vi "Operate_CSM_template_doc.vi"(6 "Save to md(F)/Load to vi(T)":bool=TRUE, 9 "Path":path=path "D:/github/JKI-State-Machine-Plus/src/help/NEVSTOP/JKI State Machine++/Template Description.md", 11 "vi path":path=path "D:/github/JKI-State-Machine-Plus/src/user.lib/_NEVSTOP/JKI State Machine++/JKISM++ No-Event Structure Template.vi") -> ()   [LabVIEW 2014]
panel:
  out "Array":cluster{refnum<vi>, "Text":string}[](array[cluster])
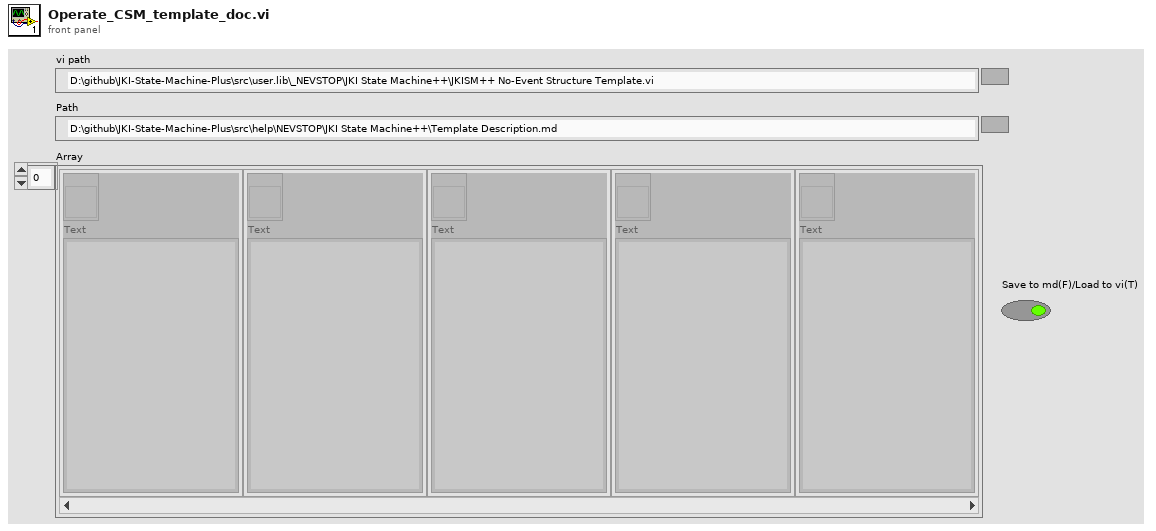
[diagram p1: front panel]
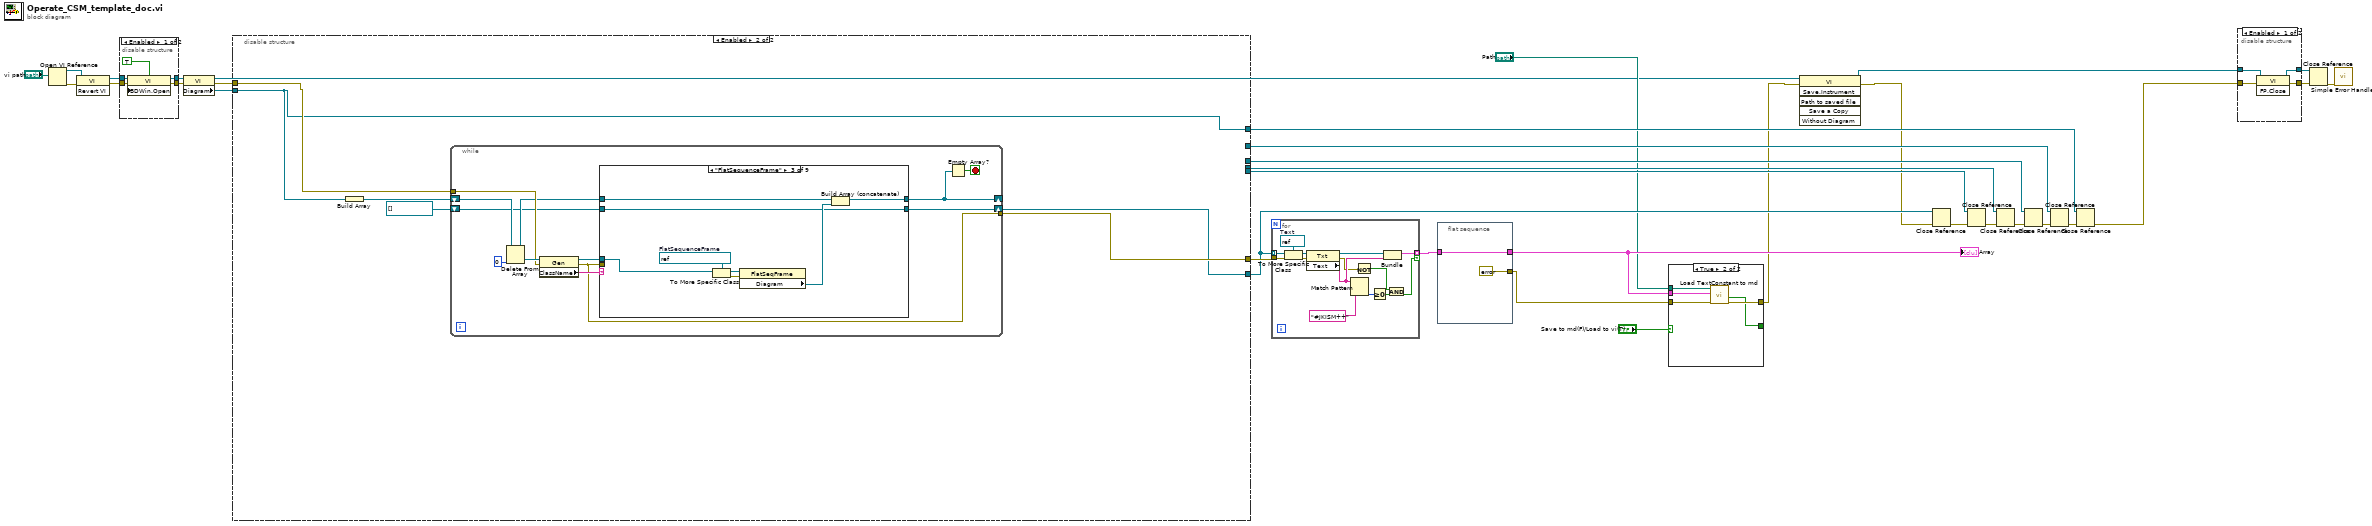
[diagram p0: block diagram]
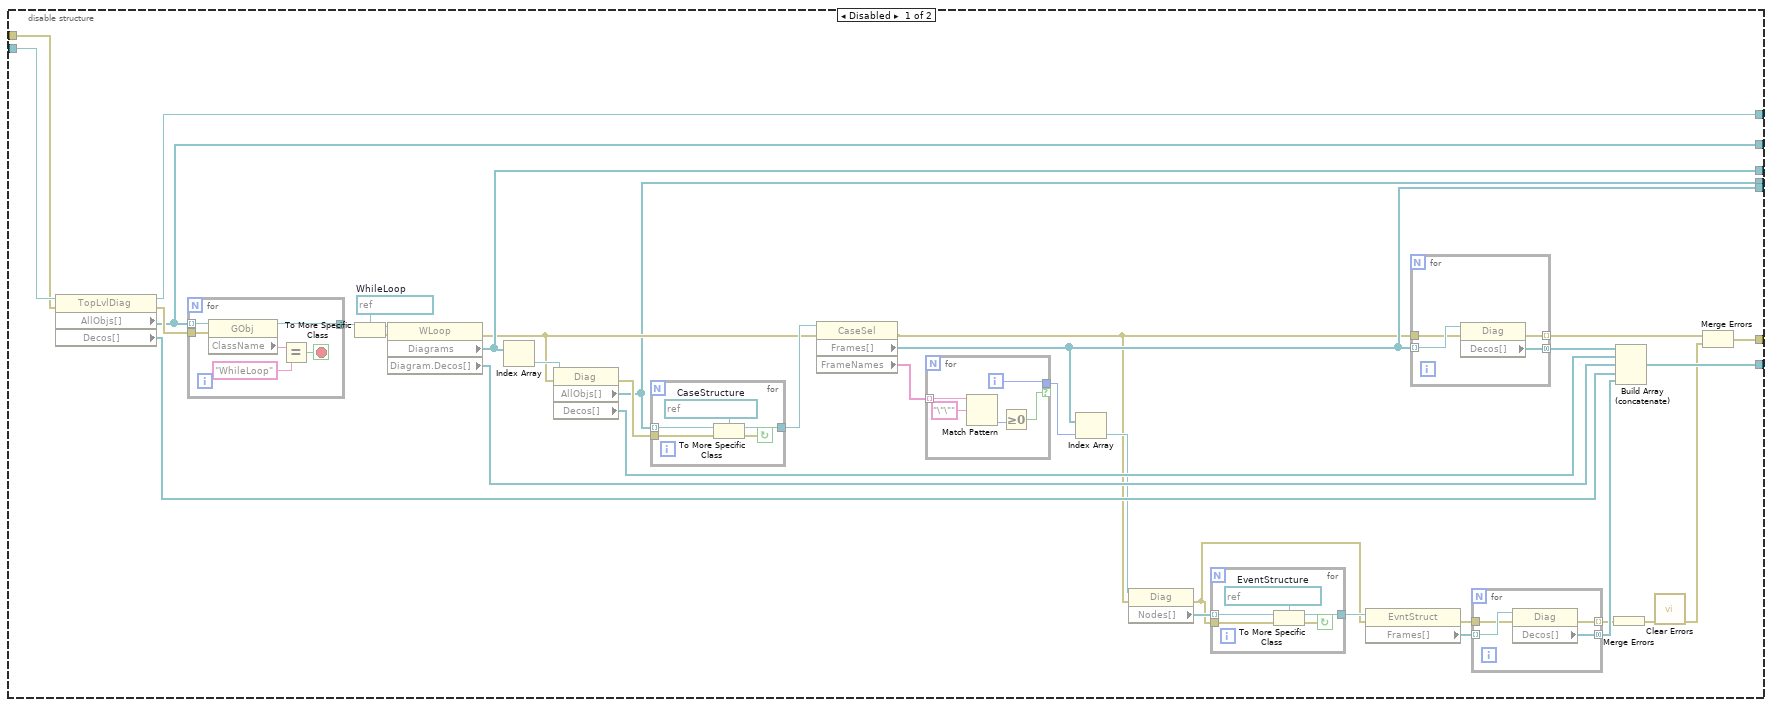
[diagram p2: hidden frame]
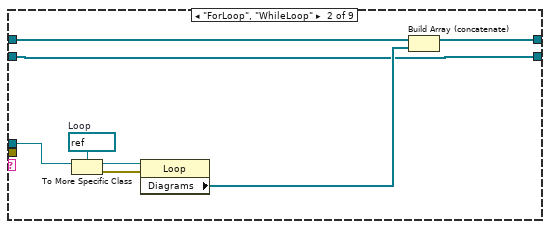
[diagram p4: hidden frame]
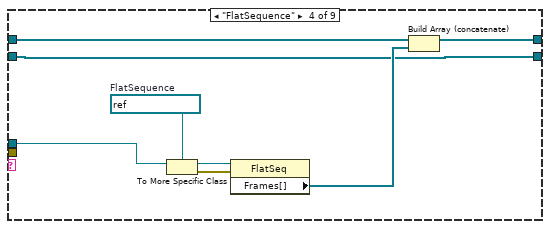
[diagram p5: hidden frame]
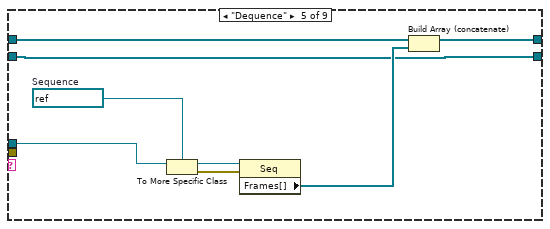
[diagram p6: hidden frame]
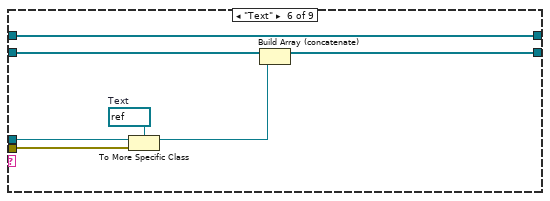
[diagram p7: hidden frame]
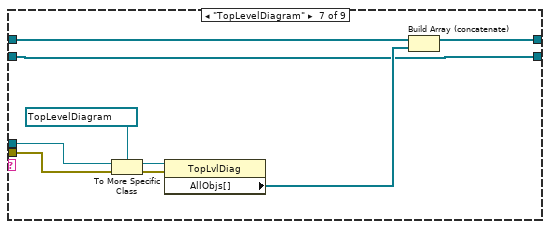
[diagram p8: hidden frame]
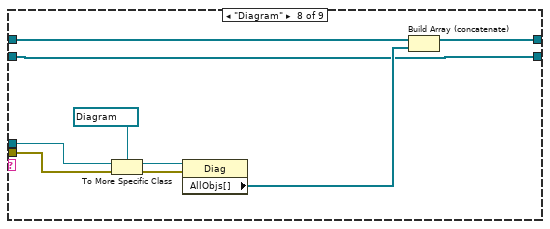
[diagram p9: hidden frame]
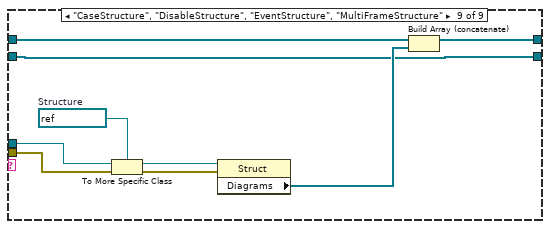
[diagram p10: hidden frame]
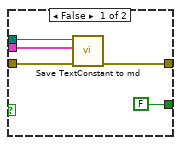
[diagram p12: hidden frame]
diagram:
  n1 = Open VI Reference(vi path="vi path") -> (vi reference=w33:refnum<vi>, error out=w34:errorcluster)  [unwired: 5 in]
  n2 = invoke class="VI" method="Revert VI"(reference=w33, error in=w34) -> (reference out=w25:refnum<vi>, error out=w24:errorcluster)  [unwired: 1 in, 1 out]
  n3 = disable-structure shown="Enabled" {
    disable-tunnel: w25 -> [w39 w41]
    disable-tunnel: w24 -> [w38 w40]
    disable-tunnel: [w37 w41] -> w23
    disable-tunnel: [w36 w40] -> w22
    frame Enabled {
      n4 = property class="VI"(reference=w39, error in=w38, "BDWin.Open"=TRUE ("Block Diagram Window:Open")) -> (reference out=w37:refnum<vi>, error out=w36:errorcluster)
    }
    frame Disabled {
    }
  }
  n5 = property class="VI"(reference=w23, error in=w22) -> (reference out=w4:refnum<vi>, error out=w30:errorcluster, "Diagram"=w31:refnum<vi>)
  n6 = disable-structure shown="Enabled" {
    disable-tunnel: w31 -> [w77 w107]
    disable-tunnel: w30 -> [w76 w110]
    disable-tunnel: [w70 _] -> w28
    disable-tunnel: [w69 w107] -> w26
    disable-tunnel: [w68 _] -> w21
    disable-tunnel: [w63 _] -> w17
    disable-tunnel: [w61 w109] -> w13
    disable-tunnel: [w58 w108] -> w12
    disable-tunnel: [w54 _] -> w11
    frame Disabled {
      w73 = refnum<vi> refnum  # WhileLoop
      n7 = property class="TopLvlDiag"(reference=w77, error in=w76) -> (reference out=w69:refnum<vi>, error out=w75:errorcluster, "AllObjs[]"=w70:refnum<vi>[], "Decos[]"=w56:refnum<vi>[])
      n8 = for {
        tunnel: w70 -> [w106] mode=indexing
        tunnel: w75 -> [w105]
        tunnel: [w104] -> w74
        stop <- w101 stop-if-true
        n9 = property class="GObj"(reference=w106, error in=w105) -> (reference out=w104:refnum<vi>, "ClassName"=w103:string)  [unwired: 1 out]
        n10 = Equal?(x=w103, y="WhileLoop") -> (x = y?=w101:bool)
      }
      n11 = To More Specific Class(target class=w73, reference=w74) -> (specific class reference=w72:refnum<vi>, error out=w71:errorcluster)  [unwired: 1 in]
      n12 = property class="WLoop"(reference=w72, error in=w71) -> (error out=w64:errorcluster, "Diagrams"=w68:refnum<vi>[], "Diagram.Decos[]"=w57:refnum<vi>[])  [unwired: 1 out]
      n13 = Index Array(array=w68) -> (element=w67:refnum<vi>)  [unwired: 1 in]
      n14 = property class="Diag"(reference=w67, error in=w64) -> (error out=w66:errorcluster, "AllObjs[]"=w63:refnum<vi>[], "Decos[]"=w59:refnum<vi>[])  [unwired: 1 out]
      n15 = for {
        tunnel: w63 -> [w100] mode=indexing
        tunnel: w66 -> [w99]
        tunnel: [w97] -> w65
        stop <- w98 continue-if-true
        w96 = refnum<vi> refnum  # CaseStructure
        n16 = To More Specific Class(target class=w96, reference=w100, error in=w99) -> (specific class reference=w97:refnum<vi>, error out=w98:errorcluster)
      }
      n17 = property class="CaseSel"(reference=w65, error in=w64) -> (error out=w45:errorcluster, "Frames[]"=w54:refnum<vi>[], "FrameNames"=w55:string[])  [unwired: 1 out]
      n18 = for {
        tunnel: w55 -> [w91] mode=indexing
        tunnel: [w89] -> w53 if=w87
        i -> [w89]
        n19 = Match Pattern(string=w91, regular expression="\"\"") -> (offset past match=w88:i32)  [unwired: 1 in, 3 out]
        n20 = Greater Or Equal To 0?(x=w88) -> (x >= 0?=w87:bool)
      }
      n21 = Index Array(array=w54, index=w53) -> (element=w52:refnum<vi>)
      n22 = property class="Diag"(reference=w52, error in=w45) -> (error out=w48:errorcluster, "Nodes[]"=w51:refnum<vi>[])  [unwired: 1 out]
      n23 = for {
        tunnel: w51 -> [w86] mode=indexing
        tunnel: w48 -> [w85]
        tunnel: [w83] -> w50
        stop <- w84 continue-if-true
        w82 = refnum<vi> refnum  # EventStructure
        n24 = To More Specific Class(target class=w82, reference=w86, error in=w85) -> (specific class reference=w83:refnum<vi>, error out=w84:errorcluster)
      }
      n25 = property class="EvntStruct"(reference=w50, error in=w48) -> (error out=w47:errorcluster, "Frames[]"=w49:refnum<vi>[])  [unwired: 1 out]
      n26 = for {
        tunnel: w54 -> [w95] mode=indexing
        tunnel: w45 -> [w94]
        tunnel: [w93] -> w62 mode=indexing
        tunnel: [w92] -> w60 mode=concatenating
        n27 = property class="Diag"(reference=w95, error in=w94) -> (error out=w93:errorcluster, "Decos[]"=w92:refnum<vi>[])  [unwired: 1 out]
      }
      n28 = for {
        tunnel: w49 -> [w81] mode=indexing
        tunnel: w47 -> [w80]
        tunnel: [w79] -> w44 mode=indexing
        tunnel: [w78] -> w46 mode=concatenating
        n29 = property class="Diag"(reference=w81, error in=w80) -> (error out=w79:errorcluster, "Decos[]"=w78:refnum<vi>[])  [unwired: 1 out]
      }
      n30 = Merge Errors(w44) -> (w43:errorcluster)
      n31 = Build Array (concatenate)(w60, w59, w57, w56, w46) -> (w58:refnum<vi>[])
      n32 = call <vilib>:"Clear Errors.vi"("error in (no error)"=w43) -> ("error out"=w42:errorcluster)  [unwired: 5 in, 1 out]
      n33 = Merge Errors(w62, w42) -> (w61:errorcluster)
    }
    frame Enabled {
      n34 = Build Array(w107) -> (w111:refnum<vi>[])
      n35 = while {
        shift-right: [w117] -> _
        shift-left: w111 -> [w123]
        shift-right: [w114] -> w108
        shift-left: refnum<vi>[] [] -> [w115]
        tunnel: w110 -> [w118]
        tunnel: [w113] -> w109
        stop <- w124 stop-if-true
        n36 = Delete From Array(array=w123, index=0) -> (deleted portion=w121:refnum<vi>, array with subset deleted=w116:refnum<vi>[])  [unwired: 1 in]
        n37 = property class="Gen"(reference=w121, error in=w118) -> (reference out=w119:refnum<vi>, error out=w113:errorcluster, "ClassName"=w120:string)
        n38 = case shown="\"FlatSequenceFrame\"" w120 {
          tunnel: w119 -> [_ w131 w139 w148 w156 w161 w172 w181 w190]
          tunnel: w113 -> [_ _ _ _ _ w162 w167 w176 w185]
          tunnel: [w126 w129 w137 w146 w154 w165 w170 w179 w188] -> w117
          tunnel: w116 -> [w126 w130 w138 w147 w155 w165 w171 w180 w189]
          tunnel: w115 -> [w125 w127 w135 w144 w152 w164 w168 w177 w186]
          tunnel: [w125 w127 w135 w144 w152 w163 w168 w177 w186] -> w114
          frame "False", Default {
          }
          frame "ForLoop", "WhileLoop" {
            w132 = refnum<vi> refnum  # Loop
            n39 = To More Specific Class(target class=w132, reference=w131) -> (specific class reference=w133:refnum<vi>, error out=w134:errorcluster)  [unwired: 1 in]
            n40 = property class="Loop"(reference=w133, error in=w134) -> ("Diagrams"=w128:refnum<vi>[])  [unwired: 2 out]
            n41 = Build Array (concatenate)(w130, w128) -> (w129:refnum<vi>[])
          }
          frame "FlatSequenceFrame" {
            w140 = refnum<vi> refnum  # FlatSequenceFrame
            n42 = To More Specific Class(target class=w140, reference=w139) -> (specific class reference=w141:refnum<vi>, error out=w142:errorcluster)  [unwired: 1 in]
            n43 = property class="FlatSeqFrame"(reference=w141, error in=w142) -> ("Diagram"=w136:refnum<vi>)  [unwired: 2 out]
            n44 = Build Array (concatenate)(w138, w136) -> (w137:refnum<vi>[])
          }
          frame "FlatSequence" {
            w143 = refnum<vi> refnum  # FlatSequence
            n45 = To More Specific Class(target class=w143, reference=w148) -> (specific class reference=w149:refnum<vi>, error out=w150:errorcluster)  [unwired: 1 in]
            n46 = property class="FlatSeq"(reference=w149, error in=w150) -> ("Frames[]"=w145:refnum<vi>[])  [unwired: 2 out]
            n47 = Build Array (concatenate)(w147, w145) -> (w146:refnum<vi>[])
          }
          frame "Dequence" {
            w151 = refnum<vi> refnum  # Sequence
            n48 = To More Specific Class(target class=w151, reference=w156) -> (specific class reference=w157:refnum<vi>, error out=w158:errorcluster)  [unwired: 1 in]
            n49 = property class="Seq"(reference=w157, error in=w158) -> ("Frames[]"=w153:refnum<vi>[])  [unwired: 2 out]
            n50 = Build Array (concatenate)(w155, w153) -> (w154:refnum<vi>[])
          }
          frame "Text" {
            w159 = refnum<vi> refnum  # Text
            n51 = To More Specific Class(target class=w159, reference=w161, error in=w162) -> (specific class reference=w160:refnum<vi>)  [unwired: 1 out]
            n52 = Build Array (concatenate)(w164, w160) -> (w163:refnum<vi>[])
          }
          frame "TopLevelDiagram" {
            n53 = To More Specific Class(target class=refnum<vi> refnum ("Block Diagram"), reference=w172, error in=w167) -> (specific class reference=w173:refnum<vi>, error out=w174:errorcluster)
            n54 = property class="TopLvlDiag"(reference=w173, error in=w174) -> ("AllObjs[]"=w169:refnum<vi>[])  [unwired: 2 out]
            n55 = Build Array (concatenate)(w171, w169) -> (w170:refnum<vi>[])
          }
          frame "Diagram" {
            n56 = To More Specific Class(target class=refnum<vi> refnum ("Block Diagram"), reference=w181, error in=w176) -> (specific class reference=w182:refnum<vi>, error out=w183:errorcluster)
            n57 = property class="Diag"(reference=w182, error in=w183) -> ("AllObjs[]"=w178:refnum<vi>[])  [unwired: 2 out]
            n58 = Build Array (concatenate)(w180, w178) -> (w179:refnum<vi>[])
          }
          frame "CaseStructure", "DisableStructure", "EventStructure", "MultiFrameStructure" {
            w184 = refnum<vi> refnum  # Structure
            n59 = To More Specific Class(target class=w184, reference=w190, error in=w185) -> (specific class reference=w191:refnum<vi>, error out=w192:errorcluster)
            n60 = property class="Struct"(reference=w191, error in=w192) -> ("Diagrams"=w187:refnum<vi>[])  [unwired: 2 out]
            n61 = Build Array (concatenate)(w189, w187) -> (w188:refnum<vi>[])
          }
        }
        n62 = Empty Array?(array=w117) -> (empty?=w124:bool)
      }
    }
  }
  n63 = for {
    tunnel: w12 -> [w206] mode=indexing
    tunnel: w13 -> [w205]
    tunnel: [w199] -> w14 mode=indexing if=w195
    w204 = refnum<vi> refnum  # Text
    n64 = To More Specific Class(target class=w204, reference=w206, error in=w205) -> (specific class reference=w203:refnum<vi>, error out=w201:errorcluster)
    n65 = property class="Txt"(reference=w203, error in=w201) -> (reference out=w202:refnum<vi>, error out=w194:errorcluster, "Text"=w198:string)
    n66 = Match Pattern(string=w198, regular expression="#JKISM++") -> (offset past match=w197:i32)  [unwired: 1 in, 3 out]
    n67 = Not(x=w194) -> (.not. x?=w193:bool)
    n68 = Greater Or Equal To 0?(x=w197) -> (x >= 0?=w196:bool)
    n69 = Bundle(w202, "Text"=w198) -> (w199:cluster{refnum<vi>, "Text":string})  [unwired: 1 in]
    n70 = And(x=w193, y=w196) -> (x .and. y?=w195:bool)
  }
  n71 = flat-sequence {
    tunnel: w14 -> [w207]
    tunnel: [errorcluster {"status"=FALSE, "code"=0, "source"=""} ("error in (no error)")] -> w9
    tunnel: [w207] -> w15
    frame #0 {
    }
  }
  n72 = case shown="True" "Save to md(F)/Load to vi(T)" {
    tunnel: w15 -> [w213 w217]
    tunnel: "Path" -> [w212 w216]
    tunnel: w9 -> [w211 w218]
    tunnel: [w210 w215] -> w3
    tunnel: [FALSE w214] -> _
    frame False {
      n73 = call "Save TextConstant to md.vi"("error in (no error) 2"=w211, "Array 2"=w213, "Path 2"=w212) -> ("error out 2"=w210:errorcluster)  [unwired: 8 in]
    }
    frame True {
      n74 = call "Load TextConstant to md.vi"("error in (no error)"=w218, "Array"=w217, "Path"=w216) -> ("error out"=w215:errorcluster, "logical AND"=w214:bool)  [unwired: 7 in]
    }
  }
  n75 = invoke class="VI" method="Save.Instrument"(reference=w4, error in=w3) -> (reference out=w6:refnum<vi>, error out=w2:errorcluster)  [unwired: 4 in, 4 out]
  n76 = Close Reference(reference=w12, error in (no error)=w2) -> (error out=w20:errorcluster)
  n77 = Close Reference(reference=w11, error in (no error)=w20) -> (error out=w19:errorcluster)
  n78 = Close Reference(reference=w17, error in (no error)=w19) -> (error out=w18:errorcluster)
  n79 = Close Reference(reference=w21, error in (no error)=w18) -> (error out=w29:errorcluster)
  n80 = Close Reference(reference=w28, error in (no error)=w29) -> (error out=w27:errorcluster)
  n81 = Close Reference(reference=w26, error in (no error)=w27) -> (error out=w1:errorcluster)
  n82 = disable-structure shown="Enabled" {
    disable-tunnel: [w222 w224] -> w7
    disable-tunnel: w6 -> [w221 w223]
    disable-tunnel: [w220 w223] -> w5
    disable-tunnel: w1 -> [w219 w224]
    frame Enabled {
      n83 = invoke class="VI" method="FP.Close"(reference=w221, error in=w219) -> (reference out=w220:refnum<vi>, error out=w222:errorcluster)  [unwired: 1 in, 1 out]
    }
    frame Disabled {
    }
  }
  n84 = Close Reference(reference=w5, error in (no error)=w7) -> (error out=w32:errorcluster)
  n85 = call <vilib>:"Simple Error Handler.vi"("error in (no error)"=w32) -> ()  [unwired: 4 in, 5 out]
  "Array" <- w15
